vi "Errors.vi"   [LabVIEW 2017, in "DSF Core.lvlib" / "Configuration Session.lvclass"]
uses:
  Configuration Session.lvclass
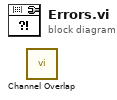
[diagram p0: block diagram]
diagram:
  n1 = call "Channel Overlap.vi"() -> ()  [unwired: 11 in, 1 out]
